vi "Check and Download Bitfile.vi"(8 "error in":errorcluster) -> (0 "error out":errorcluster)   [LabVIEW 2019, in "SEECD System Explorer.lvlib"]
uses:
  SEECD System Explorer.lvlib
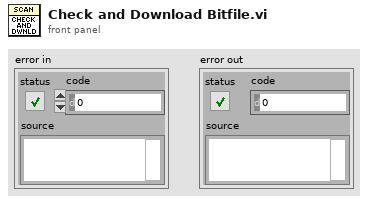
[diagram p1: front panel]
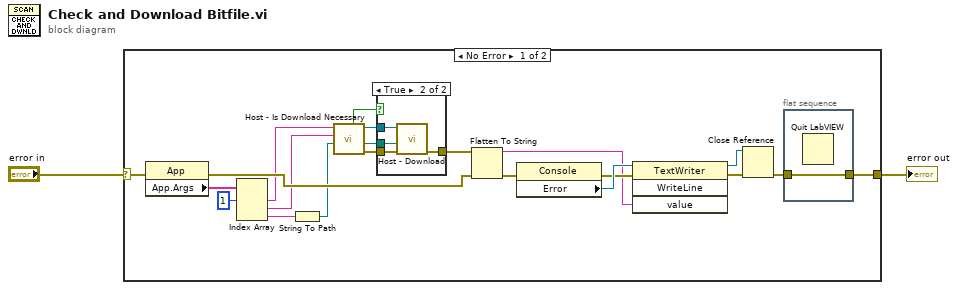
[diagram p0: block diagram]
diagram:
  n1 = case shown="No Error" "error in" {
    selector: "error in" -> [w22 w30]
    tunnel: [w20 w30] -> w1
    frame No Error {
      n2 = property class="App"(error in=w22) -> (error out=w19:errorcluster, "App.Args"=w23:string[])  [unwired: 1 in, 1 out]
      n3 = Index Array(array=w23, index #1=1 ("index")) -> (element #1=w12:string, element #2=w11:string, element #3=w18:string)  [unwired: 2 in]
      n4 = String To Path(string=w18) -> (path=w10:path)
      n5 = call "Host - Is Download Necessary.vi"("bitfile path in"=w10, "Target IP Address in"=w11, "Slave Ref in"=w12) -> ("error out"=w16:errorcluster, "bitfile path out"=w15:path, "Slave Ref out"=w14:refnum<k21>, "is download necessary?"=w17:bool)  [unwired: 4 in, 1 out]
      n6 = case shown="True" w17 {
        tunnel: w16 -> [w24 w28]
        tunnel: w15 -> [_ w27]
        tunnel: w14 -> [_ w26]
        tunnel: [w24 w25] -> w13
        frame False {
        }
        frame True {
          n7 = call "Host - Download.vi"("Error In (no error)"=w28, "bitfile path in"=w27, "Slave Ref in"=w26) -> ("error out"=w25:errorcluster)  [unwired: 6 in, 2 out]
        }
      }
      n8 = Flatten To String(anything=w13, error in (no error)=w19) -> (data string=w4:string, error out=w5:errorcluster)  [unwired: 2 in, 1 out]
      n9 = property class="Console"(error in=w5) -> (error out=w7:errorcluster, "Error"=w9:refnum<k24>)  [unwired: 1 in, 1 out]
      n10 = invoke class="TextWriter" method="WriteLine"(reference=w9, error in=w7, "value"=w4) -> (reference out=w3:refnum<k24>, error out=w8:errorcluster)  [unwired: 1 in, 2 out]
      n11 = Close Reference(reference=w3, error in (no error)=w8) -> (error out=w6:errorcluster)
      n12 = flat-sequence {
        tunnel: w6 -> [w29]
        tunnel: [w29] -> w20
        frame #0 {
          n13 = Quit LabVIEW() -> ()  [unwired: 1 in]
        }
      }
    }
    frame Error {
    }
  }
  "error out" <- w1
